vi "HP 8452 MeasSubVi.vi"(0 "GPIB in":string="18", 2 "Standard":dbl[](array[numeric]) format="%.2f", 3 "sample number":u8, 4 "setup":T2={"integration time"=0.5, "rinse time"=10.0, "sample time"=10.0, "sample type"=0} {"sample type" items=["Sample Cuvet", "Sipper Cell", "No Dialog"]; "sample time" min=0.0 max=100.0 step=1.0 format="%.1f"; "rinse time" min=0.0 max=100.0 step=1.0 format="%.1f"; "integration time" format="%.1f"}, 8 "measurement mode":T1 {"gain" max=15}) -> (5 "canceled":bool, 6 "GPIB out":string="18", 7 "measurement":dbl[](array[numeric])=[-4.07142, -4.08921, -4.05722, -4.06889, -4.04566, -4.12405, -4.10371, -4.10472, -4.01449, -4.05473, -4.09877, -3.95974, -3.98947, -3.99844, -3.98602, -3.95837, -4.10552, -4.07749, -4.0634, -4.06492, -4.08459, -4.11593, -3.97463, -4.01223, -4.04632, -4.07437, -4.09077, -4.09436, -4.08288, -4.05764, -4.02265, -3.97798, -4.11219, -4.07209, -4.03381, -4.11972, -4.10028, -4.09083, -4.09074, -4.09916, -4.11592, -4.02854, -4.05818, -4.09405, -4.12223, -3.9674, -3.98504, -3.98738, -3.984, -3.99179, -3.97789, -3.97294, -3.9582, -4.11819, -4.10696, -4.09436, -4.08184, -4.06178, -4.06657, -4.06227, -4.06236, -4.06544, -4.06669, -4.07881, -4.08798, -4.10186, -4.1157, -3.95091, -3.96565, -3.97851, -3.99177, -4.00169, -4.01187, -4.01802, -4.02114, -4.022, -4.01861, -4.01106, -4.00169, -3.98953, -3.96856, -3.94934, -4.10746, -4.08482, -4.06143, -4.0386, -4.01271, -4.12512, -4.06634, -4.11845, -4.10632, -4.10354, -4.11137, -4.12138, -4.05122, -4.05436, -4.05596, -4.05645, -4.06637, -4.08909, -4.07978, -4.12355, -4.11839, -4.12402, -4.05502, -4.0211, -4.01951, -4.04148, -4.03601, -4.03636, -4.0373, -4.05973, -4.06129, -4.05668, -4.05848, -4.09931, -3.95468, -4.10307, -4.07867, -4.09898, -3.96177, -4.06494, -4.08384, -4.0715, -4.0635, -4.07588, -4.10095, -4.08938, -4.07307, -4.04325, -4.01689, -4.10592, -4.08406, -4.07919, -4.10508, -4.07077, -4.11323, -4.08508, -4.1238, -4.06275, -4.07011, -4.09667, -4.1103, -4.09436, -4.09423, -4.11277, -4.11914, -4.10025, -4.11897, -4.07615, -4.0525, -4.10298, -4.08853, -4.10641, -4.09167, -4.0884, -4.1054, -4.1212, -4.10984, -4.1269, -4.1181, -4.09352, -4.10942, -4.10719, -4.09541, -4.10539, -4.09744, -4.10363, -4.10733, -4.08645, -4.11087, -4.10862, -4.10768, -4.10115, -4.11785, -4.10997, -4.0973, -4.10836, -4.09333, -4.12327, -4.10113, -4.12153, -4.10049, -4.10392, -4.10408, -4.1145, -4.09075, -4.06936, -4.06338, -4.04913, -4.03273, -4.05108, -3.8739, -3.90065, -3.88583, -3.95143, -3.87205, -3.88571, -4.12011, -4.07241, -3.96221, -4.12666, -4.08091, -3.97792, -4.07438, -4.07202, -4.06758, -3.97036, -4.12345, -4.0794, -4.09292, -4.06901, -4.08995, -4.11099, -4.05725, -4.09049, -4.06442, -4.09991, -4.08151, -4.11541, -4.11535, -4.11039, -4.11004, -4.11598, -4.09898, -4.12492, -4.06416, -4.05345, -4.02876, -4.09939, -4.10003, -4.11239, -4.08584, -3.95483, -4.08033, -4.08735, -4.10513, -4.0442, -3.94911, -3.94268, -4.00511, -4.09843, -3.97695, -3.99497, -4.10845, -4.10839, -4.05577, -4.09848, -4.10217, -4.1099, -4.10643, -4.11563, -4.08067, -4.11073, -4.09977, -4.01991, -4.07026, -3.99772, -4.09307, -4.11843, -4.10134, -4.08406, -4.11689, -4.04159, -4.0987, -4.09939, -4.06648, -4.10064, -4.10548, -4.12437, -4.10772, -4.12313, -4.09571, -4.11756, -4.09054, -4.1108, -4.10881, -4.10511, -4.1157, -4.12921, -4.10816, -4.10789, -4.12104, -4.0986, -4.11882, -4.1145, -4.08699, -4.1203, -4.08033, -4.09431, -4.09814, -4.12849, -4.10231, -4.07093, -4.08964, -4.12213, -4.07734, -4.12287, -4.11428, -4.10539, -4.10459, -4.09613, -4.093, -4.12292, -4.07064, -4.06091, -4.01824, -4.02458, -4.11665, -4.09893, -4.04747, -3.96943, -4.03416, -3.9858, -3.94538, -3.97187] format="%.3e")   [LabVIEW 2015]
uses:
  settings.ctl
  measurement mode.ctl
panel:
  out "Absorbance":cluster{i32, i32, dbl[]}(graph)
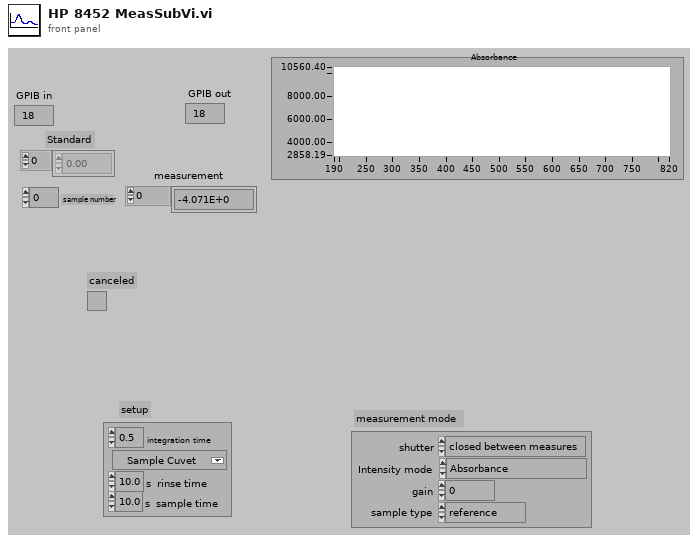
[diagram p1: front panel]
types:
  T1 = typedef "measurement mode.ctl" = cluster{"shutter":enum16{"closed between measures", "open between measures"}, "Intensity mode":enum16{"Absorbance", "Intensity at current gain", "Intensity at fixed gain", "dark current at current gain", "dark current at fixed gain"}, "gain":u8, "sample type":enum16{"reference", "standard", "unknown", "Diagnostic"}}
  T2 = typedef "settings.ctl" = cluster{"integration time":sgl, "rinse time":dbl[unit], "sample time":dbl[unit], "sample type":u16}
  T3 = enum16{"reference", "standard", "unknown", "Diagnostic"}
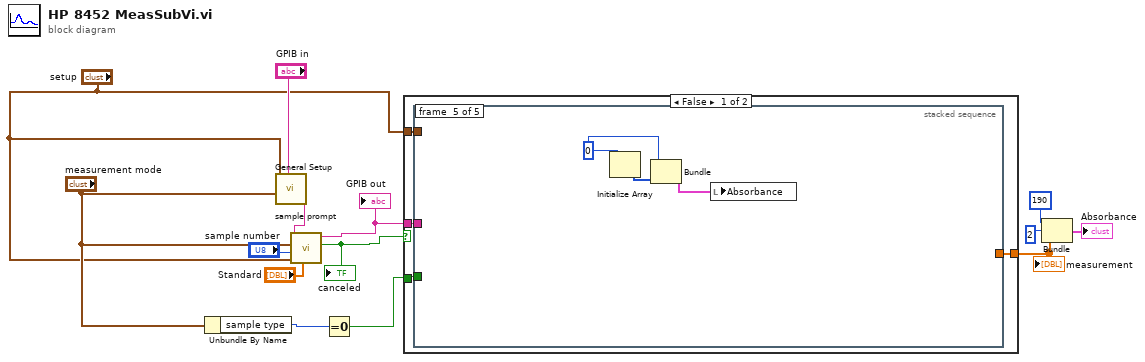
[diagram p0: block diagram]
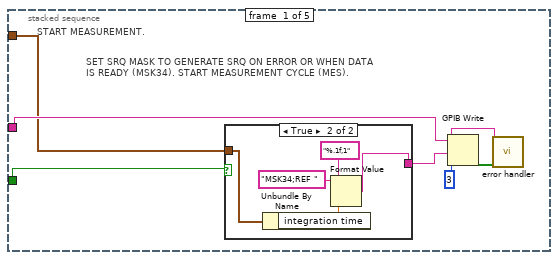
[diagram p2: hidden frame]
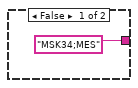
[diagram p3: hidden frame]
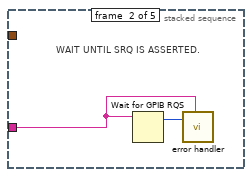
[diagram p4: hidden frame]
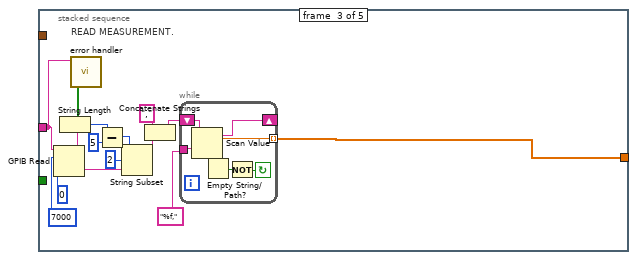
[diagram p5: hidden frame]
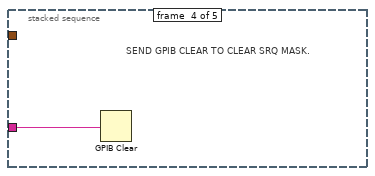
[diagram p6: hidden frame]
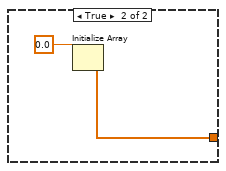
[diagram p7: hidden frame]
diagram:
  n1 = Unbundle By Name("measurement mode") -> ("sample type"=w10:T3)
  n2 = call "General Setup.vi"("measurement mode"="measurement mode", "setup"="setup", "GPIB in"="GPIB in") -> ("GPIB out"=w13:string)  [unwired: 8 in]
  n3 = call "sample prompt"("Standard"="Standard", "setup"="setup", "sample number"="sample number", "measurement mode"="measurement mode", "GPIB in"=w13) -> ("canceled"=w5:bool, "GPIB out"=w12:string)  [unwired: 3 in, 2 out]
  "GPIB out" <- w12
  "canceled" <- w5
  n4 = Equal To 0?(x=w10) -> (x = 0?=w9:bool)
  n5 = case shown="False" w5 {
    tunnel: w12 -> [w18 _]
    tunnel: "setup" -> [w17 _]
    tunnel: w9 -> [w16 _]
    tunnel: [w15 w57] -> w6
    frame False {
      n6 = stacked-sequence {
        tunnel: w18 -> [w20 w32 w34 w53 _]
        tunnel: w17 -> [w19 _ _ _ _]
        tunnel: w16 -> [w21 _ _ _ _]
        tunnel: [_ _ w33 _ _] -> w15
        frame #0 {
          # "SET SRQ MASK TO GENERATE SRQ ON ERROR OR WHEN DATA\nIS READY (MSK34). START MEASUREMENT CYCLE (MES)."
          # "START MEASUREMENT."
          n7 = case shown="True" w21 {
            tunnel: ["MSK34;MES" w27] -> w24
            tunnel: w19 -> [_ w26]
            frame False {
            }
            frame True {
              n8 = Unbundle By Name(w26) -> ("integration time"=w28:sgl)
              n9 = Format Value(string ("")="MSK34;REF ", format string="%.1f,1", value (0)=w28) -> (output string=w27:string)
            }
          }
          n10 = GPIB Write(0:w20, 1:w24, 2:3) -> (5:w22:bool[])  [unwired: 2 in, 1 out]
          n11 = call "error handler.vi"("status array"=w22, "GPIB in"=w20) -> ()  [unwired: 3 in, 3 out]
        }
        frame #1 {
          # "WAIT UNTIL SRQ IS ASSERTED."
          n12 = Wait for GPIB RQS(4:w32) -> (1:w31:i16)  [unwired: 2 in, 1 out]
          n13 = call "error handler.vi"("poll response"=w31, "GPIB in"=w32) -> ()  [unwired: 3 in, 3 out]
        }
        frame #2 {
          # "READ MEASUREMENT."
          n14 = GPIB Read(0:w34, 1:7000, 2:0) -> (5:w44:string, 6:w35:bool[])  [unwired: 2 in, 1 out]
          n15 = String Length(string=w44) -> (length=w39:i32)
          n16 = call "error handler.vi"("status array"=w35, "GPIB in"=w34) -> ()  [unwired: 3 in, 3 out]
          n17 = Subtract(x=w39, y=5) -> (x-y=w38:i32)
          n18 = String Subset(string=w44, offset (0)=2, length (rest)=w38) -> (substring=w37:string)
          n19 = Concatenate Strings(w37, ",") -> (w42:string)
          n20 = while {
            tunnel: "%f," -> [w47]
            tunnel: [w51] -> w33 mode=indexing
            shift-left: w42 -> [w50]
            shift-right: [w49] -> _
            stop <- w52 continue-if-true
            n21 = Scan Value(string=w50, format string=w47) -> (output string=w49:string, value=w51:dbl)  [unwired: 1 in]
            n22 = Empty String/Path?(string/path=w49) -> (empty?=w48:bool)
            n23 = Not(x=w48) -> (.not. x?=w52:bool)
          }
        }
        frame #3 {
          # "SEND GPIB CLEAR TO CLEAR SRQ MASK."
          n24 = GPIB Clear(3:w53) -> ()  [unwired: 1 in, 2 out]
        }
        frame #4 {
          w54 = 0
          n25 = Initialize Array(w54) -> (w56:i32[])  [unwired: 1 in]
          n26 = Bundle(w54, w54, w56) -> (w55:cluster{i32, i32, i32[]})  [unwired: 1 in]
          n27 = local write "Absorbance"(w55) -> ()
        }
      }
    }
    frame True {
      n28 = Initialize Array(0.0) -> (w57:dbl[])  [unwired: 1 in]
    }
  }
  "measurement" <- w6
  n29 = Bundle(190, 2, w6) -> (→"Absorbance":cluster{i32, i32, dbl[]})  [unwired: 1 in]
